vi "Terminal-Test-Boot.vi"(8 "error in (no error)":errorcluster caption="错误输入（无错误）") -> (0 "error out":errorcluster caption="错误输出")   [LabVIEW 2014]
uses:
  Terminal-Global-SetValues.vi
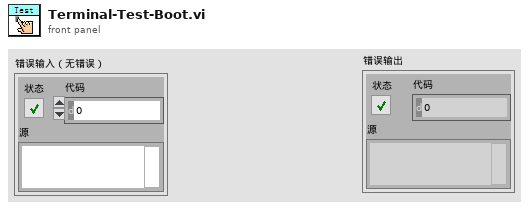
[diagram p1: front panel]
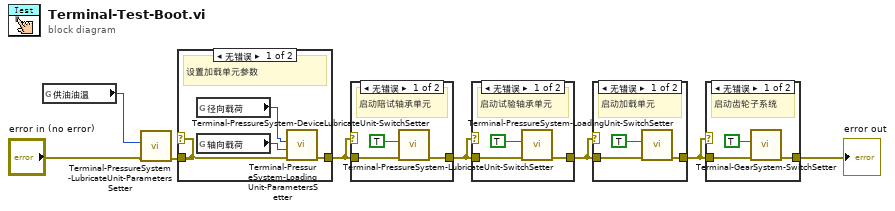
[diagram p0: block diagram]
diagram:
  n1 = global read "Terminal-Global-SetValues.vi" "供油油温"() -> (w3:u16)
  n2 = call "Terminal-PressureSystem-LubricateUnit-ParametersSetter.vi"("error in (no error)"="error in (no error)", "供油温度"=w3) -> ("error out"=w1:errorcluster)  [unwired: 9 in]
  n3 = case shown="无错误" w1 {
    tunnel: w1 -> [w11 w13]
    tunnel: [w12 w13] -> w8
    frame No Error {
      # "设置加载单元参数"
      n4 = global read "Terminal-Global-SetValues.vi" "径向载荷"() -> (w10:u16)
      n5 = global read "Terminal-Global-SetValues.vi" "轴向载荷"() -> (w9:u16)
      n6 = call "Terminal-PressureSystem-LoadingUnit-ParametersSetter.vi"("error in (no error)"=w11, "轴向液压缸加载力"=w9, "径向液压缸加载力"=w10) -> ("error out"=w12:errorcluster)  [unwired: 8 in]
    }
    frame Error {
    }
  }
  n7 = case shown="无错误" w8 {
    tunnel: w8 -> [w15 w17]
    tunnel: [w14 w17] -> w6
    frame No Error {
      # "启动陪试轴承单元"
      n8 = call "Terminal-PressureSystem-DeviceLubricateUnit-SwitchSetter.vi"("error in (no error)"=w15, "启停"=TRUE) -> ("error out"=w14:errorcluster)  [unwired: 9 in]
    }
    frame Error {
    }
  }
  n9 = case shown="无错误" w6 {
    tunnel: w6 -> [w18 w21]
    tunnel: [w19 w21] -> w5
    frame No Error {
      # "启动试验轴承单元"
      n10 = call "Terminal-PressureSystem-LubricateUnit-SwitchSetter.vi"("error in (no error)"=w18, "启停"=TRUE) -> ("error out"=w19:errorcluster)  [unwired: 9 in]
    }
    frame Error {
    }
  }
  n11 = case shown="无错误" w5 {
    tunnel: w5 -> [w22 w25]
    tunnel: [w23 w25] -> w4
    frame No Error {
      # "启动加载单元"
      n12 = call "Terminal-PressureSystem-LoadingUnit-SwitchSetter.vi"("error in (no error)"=w22, "启停"=TRUE) -> ("error out"=w23:errorcluster)  [unwired: 9 in]
    }
    frame Error {
    }
  }
  n13 = case shown="无错误" w4 {
    tunnel: w4 -> [w28 w29]
    tunnel: [w27 w29] -> w7
    frame No Error {
      # "启动齿轮子系统"
      n14 = call "Terminal-GearSystem-SwitchSetter.vi"("error in (no error)"=w28, "启停"=TRUE) -> ("error out"=w27:errorcluster)  [unwired: 9 in]
    }
    frame Error {
    }
  }
  "error out" <- w7
